vi "Run Batch file As Admin.vi"(8 "error in (no error)":errorcluster, 11 "BAT File Content":string) -> (0 "error out":errorcluster)   [LabVIEW 2022 SP3, in "NIPM_Functions.lvlib"]
uses:
  NIPM_Functions.lvlib
  shell32.dll
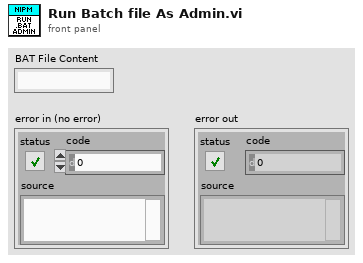
[diagram p1: front panel]
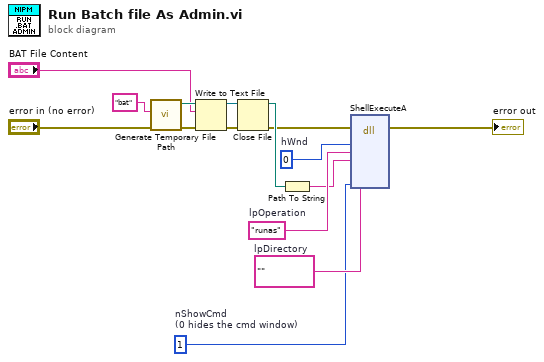
[diagram p0: block diagram]
diagram:
  w14 = 1  # nShowCmd (0 hides the cmd window)
  w15 = ""  # lpDirectory
  w13 = "runas"  # lpOperation
  w12 = 0  # hWnd
  n1 = call <vilib>:"Generate Temporary File Path.vi"("error in (no error)"="error in (no error)", "Temporary File Extension (tmp)"="bat") -> ("error out"=w9:errorcluster, "Unique Temporary File Path"=w8:path)  [unwired: 8 in]
  n2 = Write to Text File(file (use dialog)=w8, text="BAT File Content", error in=w9) -> (refnum out=w6:refnum<file>, error out=w5:errorcluster)  [unwired: 1 in, 1 out]
  n3 = Close File(refnum=w6, error in=w5) -> (path=w4:path, error out=w1:errorcluster)
  n4 = Path To String(path=w4) -> (string=w11:string)
  n5 = dll-call lib="shell32.dll" fn="ShellExecuteA"(error in=w1, "hWnd"=w12, "lpOperation"=w13, "lpFile"=w11, "lpParameters"=w15, "lpDirectory"=w15, "nShowCmd"=w14) -> (error out=→"error out":errorcluster)  [unwired: 9 in, 1 out]
